vi "Generator Lesson 5.vi"() -> ()   [LabVIEW 2019]
uses:
  <vilib>/Instr/_visa.llb/VISA Configure Serial Port (Instr).vi
  <vilib>/addons/control/pid/pid.llb/PID (DBL).vi
  <vilib>/addons/control/pid/NI_PID_pid.lvlib
panel:
  in  "stop":bool
  out "Meter":dbl(knob) scale=0.0..255.0
  out "Waveform Chart":cluster{"Setpoint":dbl, dbl}(graph)
  in  "Setpoint":dbl(slide) scale=0.0..200.0
  in  "PID gains":T1={"proportional gain (Kc)"=1.0, "integral time (Ti, min)"=0.01, "derivative time (Td, min)"=0.0} {"derivative time (Td, min)" format="%.3f"; "integral time (Ti, min)" format="%.3f"; "proportional gain (Kc)" format="%.3f"}
  in  "generator":refnum<visa-resource-name>
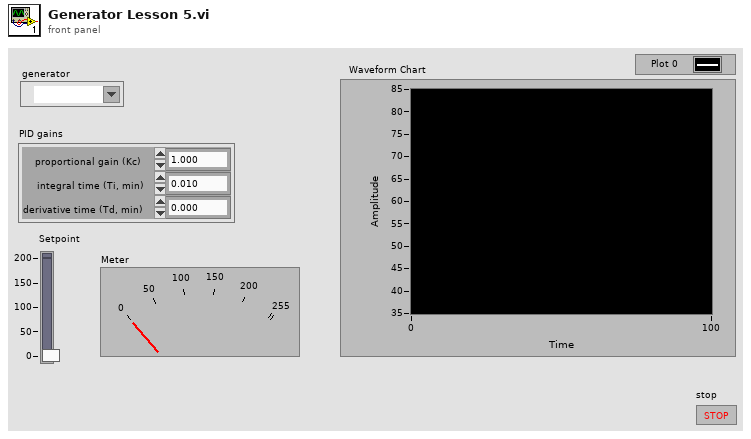
[diagram p1: front panel]
types:
  T1 = cluster{"proportional gain (Kc)":dbl, "integral time (Ti, min)":dbl, "derivative time (Td, min)":dbl}
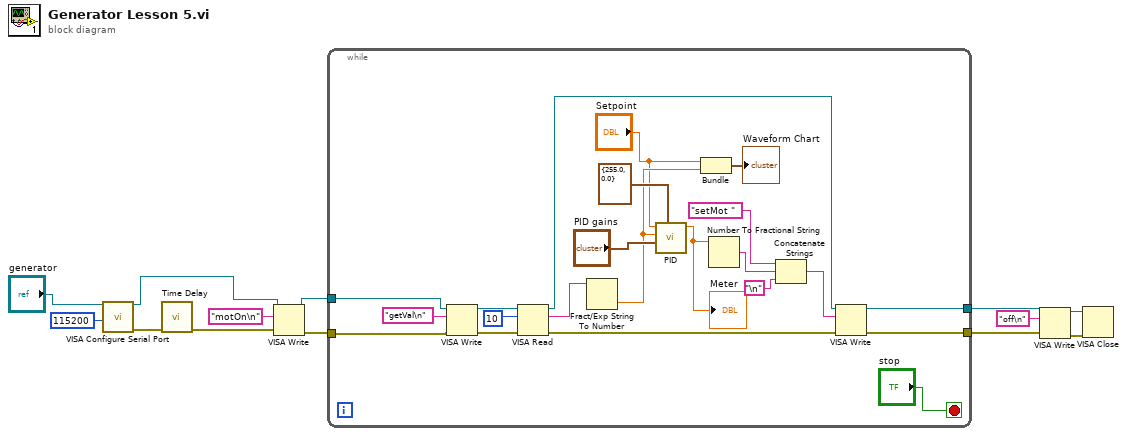
[diagram p0: block diagram]
diagram:
  n1 = call-poly "VISA Configure Serial Port"("VISA resource name"="generator", "baud rate (9600)"=u32 115200) -> ("VISA resource name out"=w9:refnum<visa-resource-name>, "error out"=w11:errorcluster)  [unwired: 12 in]
  n2 = call "Time Delay"("error in (no error)"=w11) -> ("error out"=w10:errorcluster)  [unwired: 10 in]
  n3 = VISA Write(VISA resource name=w9, write buffer="motOn\n", error in (no error)=w10) -> (VISA resource name out=w7:refnum<visa-resource-name>, error out=w1:errorcluster)  [unwired: 1 out]
  n4 = while {
    tunnel: w7 -> [w15]
    tunnel: w1 -> [w16]
    tunnel: [w24] -> w6
    tunnel: [w23] -> w5
    stop <- "stop" stop-if-true
    n5 = VISA Write(VISA resource name=w15, write buffer="getVal\n", error in (no error)=w16) -> (VISA resource name out=w35:refnum<visa-resource-name>, error out=w34:errorcluster)  [unwired: 1 out]
    n6 = VISA Read(VISA resource name=w35, byte count=u32 10, error in (no error)=w34) -> (VISA resource name out=w25:refnum<visa-resource-name>, read buffer=w33:string, error out=w26:errorcluster)  [unwired: 1 out]
    n7 = Fract/Exp String To Number(string=w33) -> (number=w22:dbl)  [unwired: 3 in, 1 out]
    n8 = call-poly <vilib>:"PID.vi"("output range"=cluster{"output high":dbl, "output low":dbl} {"output high"=255.0, "output low"=0.0}, "PID gains"="PID gains", "process variable"=w22, "setpoint"="Setpoint") -> ("output"=w19:dbl)  [unwired: 6 in, 1 out]
    "Meter" <- w19
    n9 = Bundle("Setpoint"="Setpoint", w22) -> (→"Waveform Chart":cluster{"Setpoint":dbl, dbl})  [unwired: 1 in]
    n10 = Number To Fractional String(number=w19) -> (F-format string=w29:string)  [unwired: 3 in]
    n11 = Concatenate Strings("setMot " ("string"), w29, "\n") -> (w27:string)
    n12 = VISA Write(VISA resource name=w25, write buffer=w27, error in (no error)=w26) -> (VISA resource name out=w24:refnum<visa-resource-name>, error out=w23:errorcluster)  [unwired: 1 out]
  }
  n13 = VISA Write(VISA resource name=w6, write buffer="off\n", error in (no error)=w5) -> (VISA resource name out=w4:refnum<visa-resource-name>, error out=w3:errorcluster)  [unwired: 1 out]
  n14 = VISA Close(VISA resource name=w4, error in (no error)=w3) -> ()  [unwired: 1 out]
